vi "Sell.vi"(8 "error in (no error)":errorcluster, 11 "Data cluster":T1) -> (0 "error out":errorcluster)   [LabVIEW 2020, in "Productos.lvlib"]
uses:
  Productos.lvlib
  Coins/Coins.lvlib
  Messages/Messages.lvlib
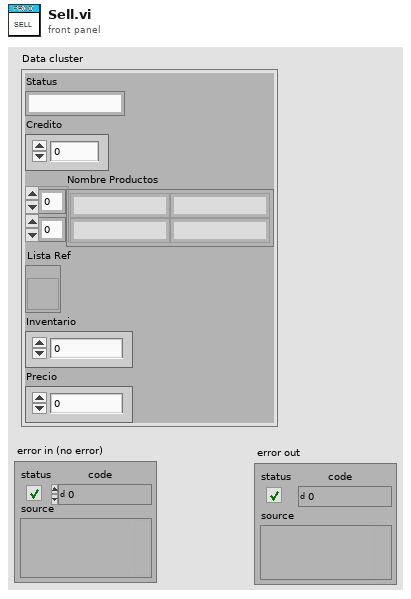
[diagram p1: front panel]
types:
  T1 = cluster{"Status":string, "Credito":dbl, "Nombre Productos":string[][], "Lista Ref":refnum<vi>, "Inventario":dbl, "Precio":dbl}
  T2 = typedef "Coins.lvlib/Request money (Reply Payload)--cluster.ctl" = cluster{"Credit":dbl, "Request money_error":errorcluster}
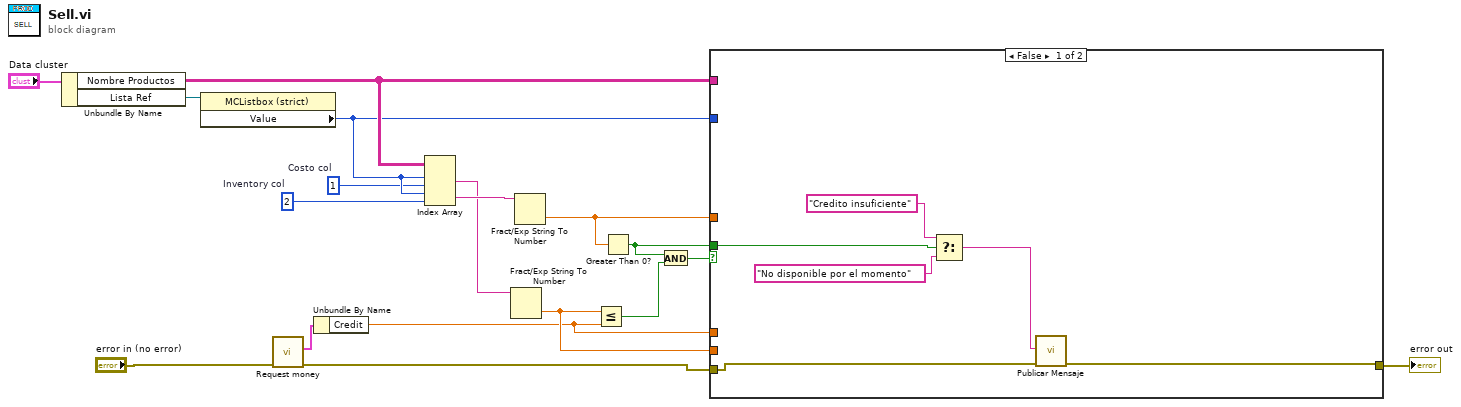
[diagram p0: block diagram]
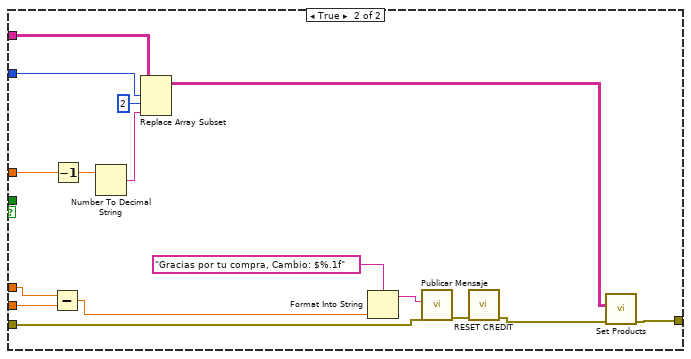
[diagram p2: hidden frame]
diagram:
  w13 = 2  # Inventory col
  w14 = 1  # Costo col
  n1 = Unbundle By Name("Data cluster") -> ("Nombre Productos"=w16:string[][], "Lista Ref"=w17:refnum<vi>)
  n2 = property class="MCListbox (strict)"(reference=w17) -> ("Value"=w15:i32)  [unwired: 1 in, 2 out]
  n3 = call "Request money.vi"("error in (no error)"="error in (no error)") -> ("error out"=w1:errorcluster, "Reply Payload"=w5:T2)  [unwired: 8 in, 1 out]
  n4 = Unbundle By Name(w5) -> ("Credit"=w3:dbl)
  n5 = Index Array(array=w16, index (row) #1=w15, index (col) #1=w14, index (row) #2=w15, index (col) #2=w13) -> (element #1=w7:string, element #2=w12:string)
  n6 = Fract/Exp String To Number(string=w7) -> (number=w4:dbl)  [unwired: 3 in, 1 out]
  n7 = Fract/Exp String To Number(string=w12) -> (number=w11:dbl)  [unwired: 3 in, 1 out]
  n8 = Less Or Equal?(x=w4, y=w3) -> (x <= y?=w8:bool)
  n9 = Greater Than 0?(x=w11) -> (x > 0?=w9:bool)
  n10 = And(x=w9, y=w8) -> (x .and. y?=w10:bool)
  n11 = case shown="False" w10 {
    tunnel: w16 -> [_ w36]
    tunnel: w15 -> [_ w34]
    tunnel: w11 -> [_ w38]
    tunnel: w9 -> [w24 _]
    tunnel: w4 -> [_ w40]
    tunnel: w3 -> [_ w39]
    tunnel: [w20 w32] -> w2
    tunnel: w1 -> [w21 w28]
    frame False {
      n12 = Select(t="Credito insuficiente", s=w24, f="No disponible por el momento") -> (s? t:f=w19:string)
      n13 = call "Publicar Mensaje.vi"("error in (no error)"=w21, "Mensaje"=w19) -> ("error out"=w20:errorcluster)  [unwired: 9 in]
    }
    frame True {
      n14 = Subtract(x=w39, y=w40) -> (x-y=w30:dbl)
      n15 = Decrement(x=w38) -> (x-1=w37:dbl)
      n16 = Number To Decimal String(number=w37) -> (decimal integer string=w35:string)  [unwired: 1 in]
      n17 = Replace Array Subset(array=w36, new element=w35, index (row)=w34, index (col)=2 ("disabled index (col)")) -> (w31:string[][])
      n18 = Format Into String(format string="Gracias por tu compra, Cambio: $%.1f", w30) -> (resulting string=w27:string)  [unwired: 2 in, 1 out]
      n19 = call "Publicar Mensaje.vi"("error in (no error)"=w28, "Mensaje"=w27) -> ("error out"=w26:errorcluster)  [unwired: 9 in]
      n20 = call "RESET CREDIT.vi"("error in (no error)"=w26) -> ("error out"=w25:errorcluster)  [unwired: 10 in]
      n21 = call "Set Products.vi"("error in (no error)"=w25, "Array"=w31) -> ("error out"=w32:errorcluster)  [unwired: 9 in]
    }
  }
  "error out" <- w2
